vi "calibrate.vi"() -> ()   [LabVIEW 2019, in "Nano33BLE-TiltCompensationSupport.lvlib"]
uses:
  types/xyz.ctl
  types/calibrate_data.ctl
  types/xyz_array.ctl
  <vilib>/Instr/_visa.llb/VISA Configure Serial Port (Instr).vi
  Nano33BLE-TiltCompensationSupport.lvlib
  <vilib>/gmath/NI_Gmath.lvlib
panel:
  out "effective calib.":T2
  out "instructions":string
  in  "mode":bool=TRUE
  out "new config":string
  in  "initial config":string="#define OFFSET_MAG_X 0.00\n#define OFFSET_MAG_Y 0.00\n#define OFFSET_MAG_Z 0.00\n#define R_MAG 1.00\n\n#define OFFSET_ACC_X 0.00\n#define OFFSET_ACC_Y 0.00\n#define OFFSET_ACC_Z 0.00\n#define R_ACC 1.00\n\n#define OFFSET_GYR_X 0.00\n#define OFFSET_GYR_Y 0.00\n#define OFFSET_GYR_Z 0.00" caption="initial config (paste from compass-support.h)"
  in  "reset?":bool
  out "acc":cluster{dbl[], dbl[]}[](graph)
  out "mag":cluster{dbl[], dbl[]}[](graph)
  out "rates":cluster{"mag":dbl, "acc":dbl, "gyr":dbl} {"mag" format="%0.1f Hz"; "acc" format="%0.1f Hz"; "gyr" format="%0.1f Hz"}
  in  "port":refnum<visa-resource-name>="COM3"
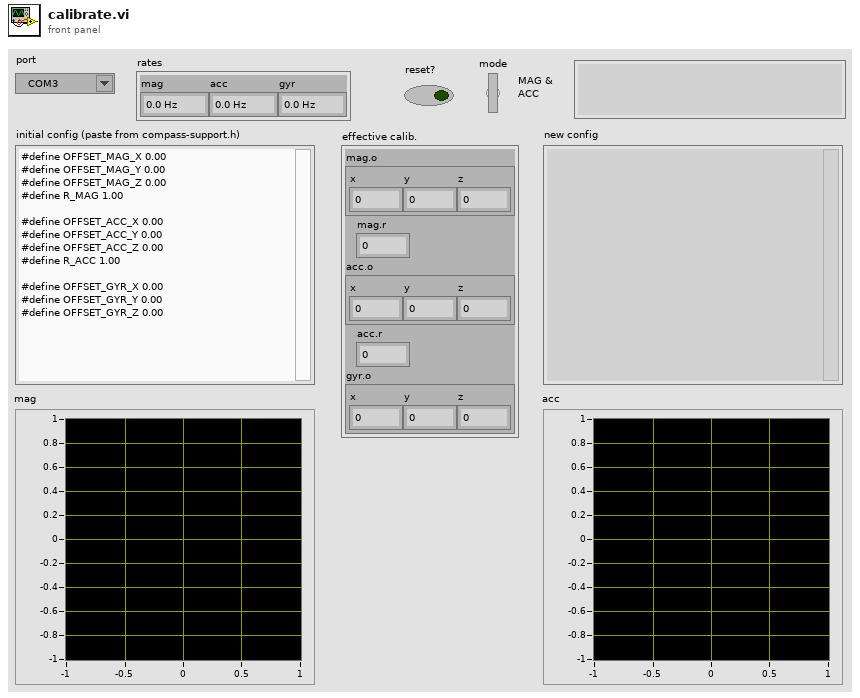
[diagram p1: front panel]
types:
  T1 = typedef "Nano33BLE-TiltCompensationSupport.lvlib/xyz.ctl" = cluster{"x":dbl, "y":dbl, "z":dbl}
  T2 = cluster{"mag.o":T1, "mag.r":dbl, "acc.o":T1, "acc.r":dbl, "gyr.o":T1}
  T3 = typedef "Nano33BLE-TiltCompensationSupport.lvlib/calibrate_data.ctl" = cluster{"mag":T4, "acc":T4, "gyr":T4, "rates":cluster{"mag":dbl, "acc":dbl, "gyr":dbl}}
  T4 = typedef "Nano33BLE-TiltCompensationSupport.lvlib/xyz_array.ctl" = cluster{"X":dbl[], "Y":dbl[], "Z":dbl[]}
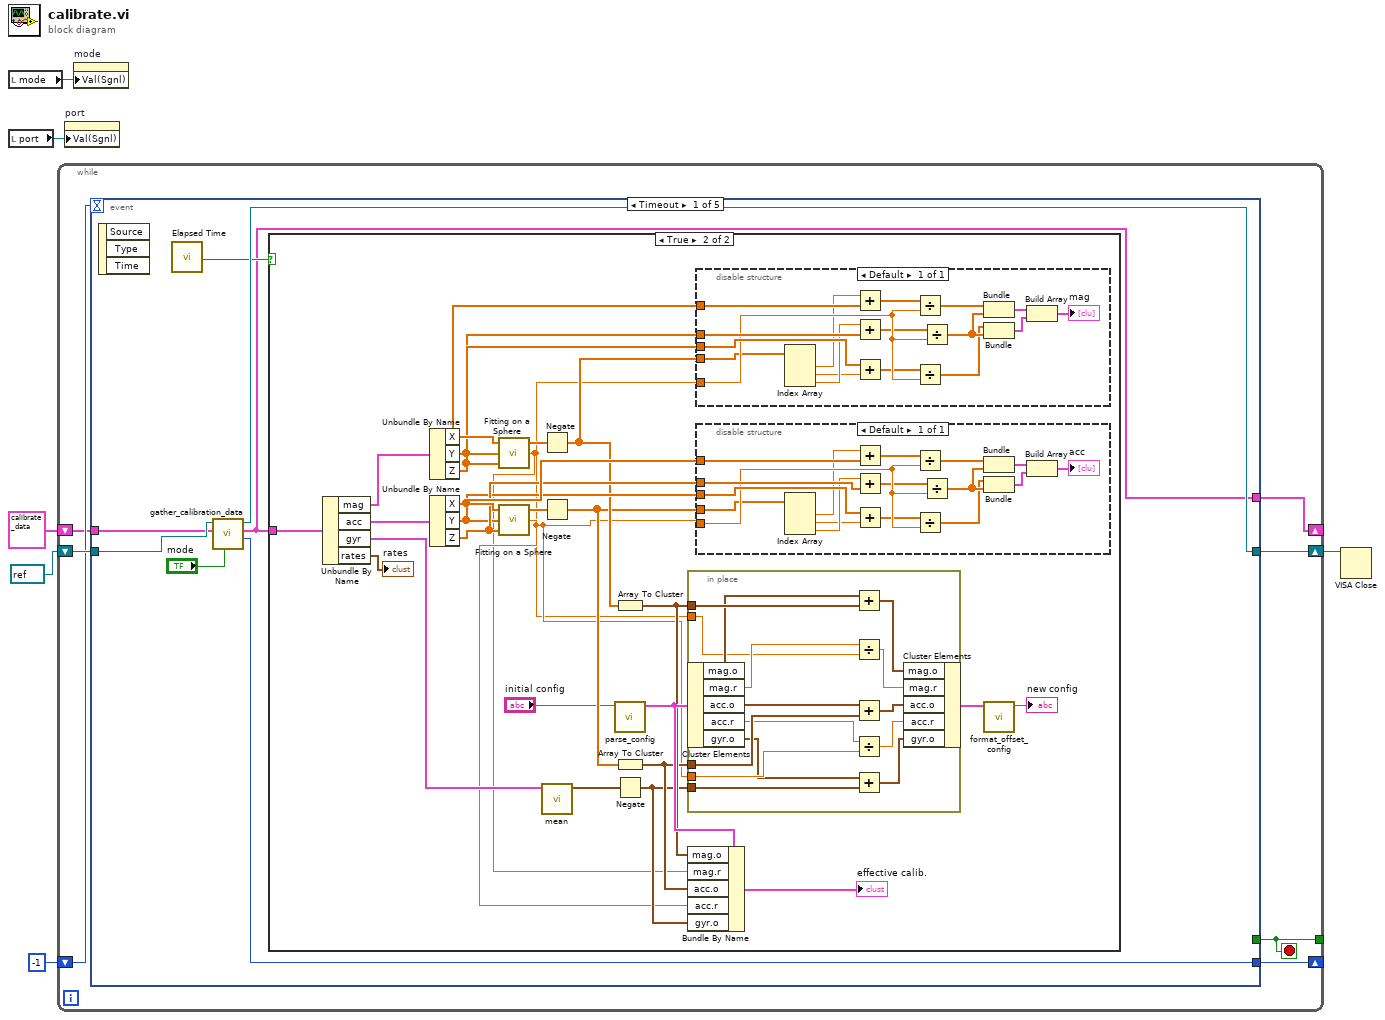
[diagram p0: block diagram]
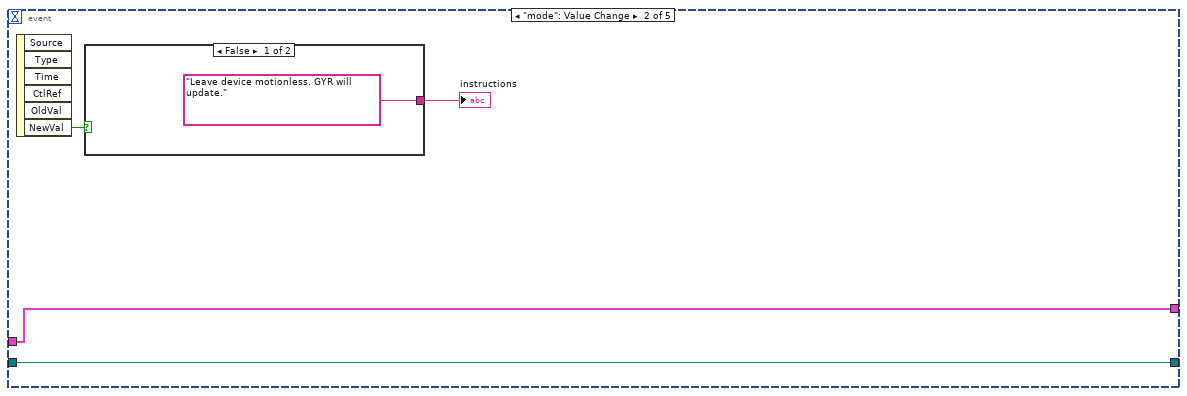
[diagram p3: hidden frame]
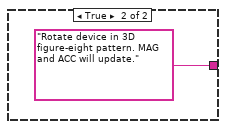
[diagram p4: hidden frame]
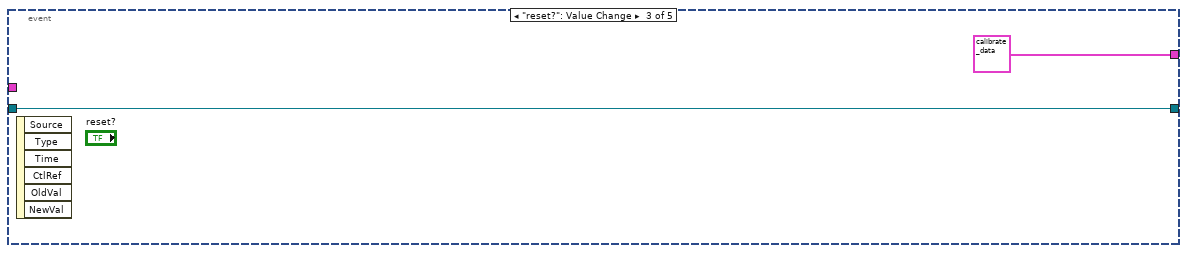
[diagram p5: hidden frame]
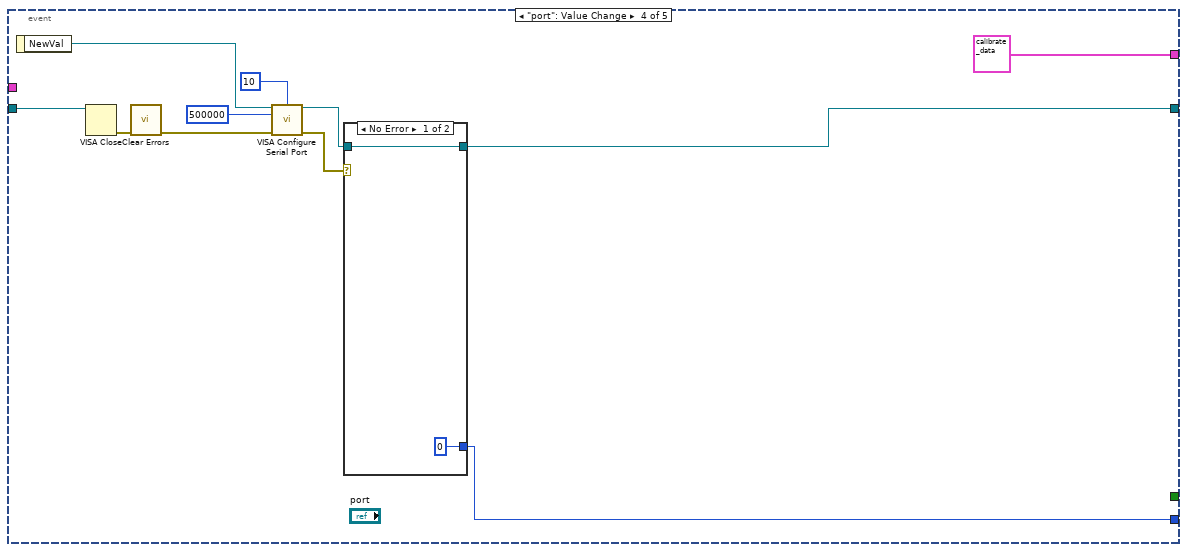
[diagram p6: hidden frame]
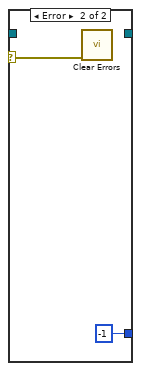
[diagram p7: hidden frame]
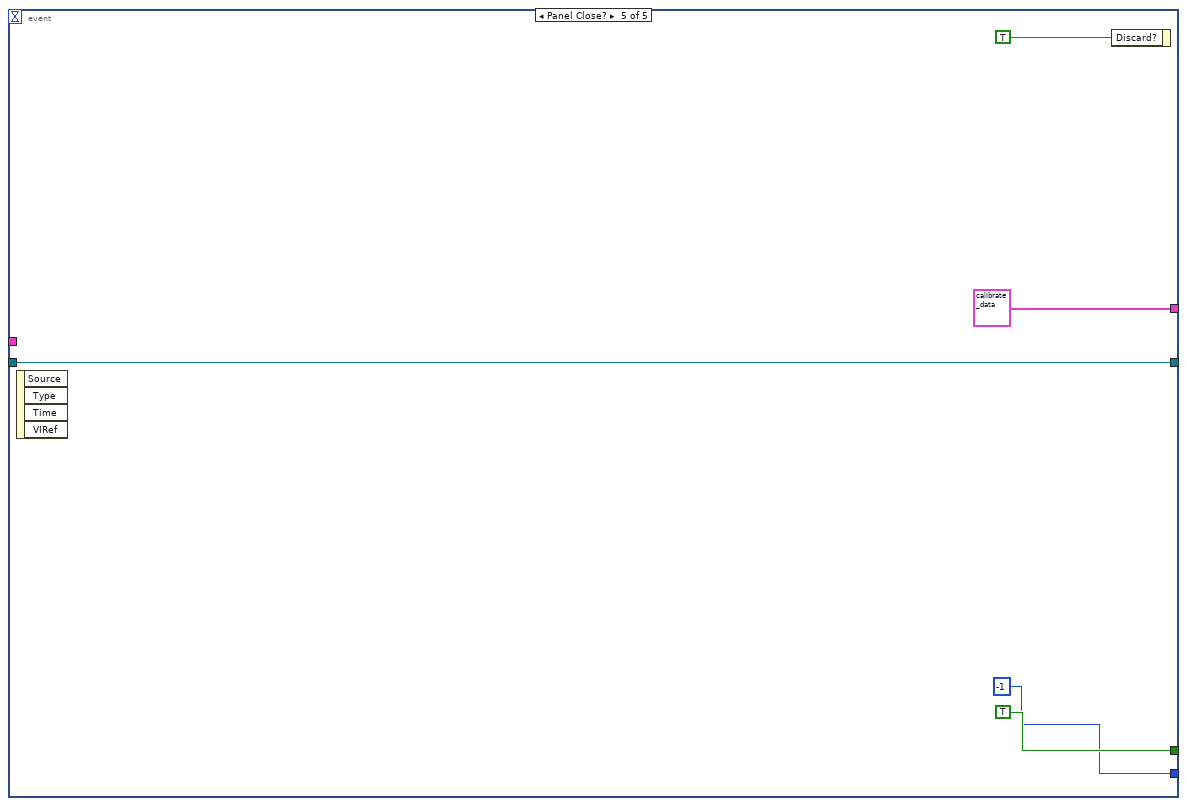
[diagram p8: hidden frame]
diagram:
  n1 = local read "mode"() -> (w1:bool)
  n2 = local read "port"() -> (w2:refnum<visa-resource-name>)
  n3 = while {
    tunnel: [w12] -> _
    shift-right: [w8] -> w3
    shift-left: refnum<visa-resource-name> refnum ("VISA resource name out") -> [w13]
    shift-right: [w9] -> _
    shift-left: -1 -> [w11]
    shift-right: [w7] -> _
    shift-left: T3 {"mag"={"X"=[], "Y"=[], "Z"=[]}, "acc"={"X"=[], "Y"=[], "Z"=[]}, "gyr"={"X"=[], "Y"=[], "Z"=[]}, "rates"={"mag"=0.0, "acc"=0.0, "gyr"=0.0}} ("data") -> [w10]
    stop <- w12 stop-if-true
    n4 = event shown="[0] Timeout" {
      selector: _ -> [_ _ _ _ _]
      dyn-events: _ -> [_ _ _ _ _]
      timeout: w11 -> [_ _ _ _ _]
      tunnel: w13 -> [w20 w96 w102 w112 w119]
      tunnel: [_ _ _ _ TRUE ("Discard?")] -> w12
      tunnel: w10 -> [w17 w99 _ _ _]
      tunnel: [w19 _ _ w108 -1] -> w9
      tunnel: [w18 w96 w102 w107 w119] -> w8
      tunnel: [w15 w99 T3 {"mag"={"X"=[], "Y"=[], "Z"=[]}, "acc"={"X"=[], "Y"=[], "Z"=[]}, "gyr"={"X"=[], "Y"=[], "Z"=[]}, "rates"={"mag"=0.0, "acc"=0.0, "gyr"=0.0}} ("data") T3 {"mag"={"X"=[], "Y"=[], "Z"=[]}, "acc"={"X"=[], "Y"=[], "Z"=[]}, "gyr"={"X"=[], "Y"=[], "Z"=[]}, "rates"={"mag"=0.0, "acc"=0.0, "gyr"=0.0}} ("data") T3 {"mag"={"X"=[], "Y"=[], "Z"=[]}, "acc"={"X"=[], "Y"=[], "Z"=[]}, "gyr"={"X"=[], "Y"=[], "Z"=[]}, "rates"={"mag"=0.0, "acc"=0.0, "gyr"=0.0}} ("data")] -> w7
      event Timeout {
        n5 = event-data() -> ()  [unwired: 1 in, 3 out]
        n6 = call "Elapsed Time"() -> ("Time has Elapsed"=w16:bool)  [unwired: 12 in, 7 out]
        n7 = call "gather_calibration_data.vi"("mode"="mode", "data in"=w17, "VISA Refnum in"=w20) -> ("next timeout (ms)"=w19:i32, "data out"=w15:T3, "VISA Refnum out"=w18:refnum<visa-resource-name>)  [unwired: 6 in]
        n8 = case shown="True" w16 {
          tunnel: w15 -> [_ w46]
          frame False {
          }
          frame True {
            n9 = Unbundle By Name(w46) -> ("mag"=w43:T4, "acc"=w42:T4, "gyr"=w45:T4, "rates"=→"rates":cluster{"mag":dbl, "acc":dbl, "gyr":dbl})
            n10 = Unbundle By Name(w43) -> ("X"=w41:dbl[], "Y"=w40:dbl[], "Z"=w39:dbl[])
            n11 = Unbundle By Name(w42) -> ("X"=w38:dbl[], "Y"=w36:dbl[], "Z"=w37:dbl[])
            n12 = call <vilib>:"Fitting on a Sphere.vi"("Z"=w39, "Y"=w40, "X"=w41) -> ("r"=w22:dbl, "x0, y0, z0"=w34:dbl[])  [unwired: 1 out]
            n13 = call <vilib>:"Fitting on a Sphere.vi"("Z"=w37, "Y"=w36, "X"=w38) -> ("r"=w23:dbl, "x0, y0, z0"=w32:dbl[])  [unwired: 1 out]
            n14 = Negate(x=w34) -> (-x=w33:dbl[])
            n15 = Negate(x=w32) -> (-x=w31:dbl[])
            n16 = call "mean.vi"("data in"=w45) -> ("xyz"=w35:T1)  [unwired: 10 in]
            n17 = Array To Cluster(array=w33) -> (cluster=w26:cluster{"[0]":dbl, "[1]":dbl, "[2]":dbl})
            n18 = call "parse_config.vi"("initial config"="initial config") -> ("config"=w27:T2)  [unwired: 10 in]
            n19 = Array To Cluster(array=w31) -> (cluster=w25:cluster{"[0]":dbl, "[1]":dbl, "[2]":dbl})
            n20 = Negate(x=w35) -> (-x=w24:T1)
            n21 = in-place {
              in-place-border: w26 -> [w61]
              in-place-border: w22 -> [w49]
              in-place-border: w25 -> [w57]
              in-place-border: w23 -> [w56]
              in-place-border: w24 -> [w52]
              n22 = in-place-cluster #1(w27) -> ("mag.o"=w50:T1, "mag.r"=w59:dbl, "acc.o"=w48:T1, "acc.r"=w47:dbl, "gyr.o"=w53:T1)
              n23 = Add(x=w50, y=w61) -> (x+y=w60:T1)
              n24 = Divide(x=w59, y=w49) -> (x/y=w58:dbl)
              n25 = Add(x=w48, y=w57) -> (x+y=w55:T1)
              n26 = Divide(x=w47, y=w56) -> (x/y=w54:dbl)
              n27 = Add(x=w53, y=w52) -> (x+y=w51:T1)
              n28 = in-place-cluster #1("mag.o"=w60, "mag.r"=w58, "acc.o"=w55, "acc.r"=w54, "gyr.o"=w51) -> (w29:T2)
            }
            n29 = Bundle By Name(cluster=w27, "mag.o"=w26, "mag.r"=w22, "acc.o"=w25, "acc.r"=w23, "gyr.o"=w24) -> (→"effective calib.":T2)
            n30 = disable-structure shown="Default" {
              disable-tunnel: w41 -> [w95]
              disable-tunnel: w40 -> [w94]
              disable-tunnel: w39 -> [w93]
              disable-tunnel: w22 -> [w92]
              disable-tunnel: w33 -> [w85]
              frame Enabled {
                n31 = Index Array(array=w85) -> (element #1=w81:dbl, element #2=w79:dbl, element #3=w80:dbl)  [unwired: 3 in]
                n32 = Add(x=w81, y=w95) -> (x+y=w84:dbl[])
                n33 = Add(x=w80, y=w93) -> (x+y=w83:dbl[])
                n34 = Add(x=w94, y=w79) -> (x+y=w82:dbl[])
                n35 = Divide(x=w84, y=w92) -> (x/y=w89:dbl[])
                n36 = Divide(x=w82, y=w92) -> (x/y=w90:dbl[])
                n37 = Divide(x=w83, y=w92) -> (x/y=w91:dbl[])
                n38 = Bundle(w89, w91) -> (w87:cluster{dbl[], dbl[]})  [unwired: 1 in]
                n39 = Bundle(w90, w91) -> (w88:cluster{dbl[], dbl[]})  [unwired: 1 in]
                n40 = Build Array(w87, w88) -> (→"mag":cluster{dbl[], dbl[]}[])
              }
            }
            n41 = disable-structure shown="Default" {
              disable-tunnel: w38 -> [w78]
              disable-tunnel: w36 -> [w77]
              disable-tunnel: w37 -> [w76]
              disable-tunnel: w23 -> [w75]
              disable-tunnel: w31 -> [w68]
              frame Enabled {
                n42 = Index Array(array=w68) -> (element #1=w64:dbl, element #2=w62:dbl, element #3=w63:dbl)  [unwired: 3 in]
                n43 = Add(x=w64, y=w78) -> (x+y=w67:dbl[])
                n44 = Add(x=w63, y=w76) -> (x+y=w66:dbl[])
                n45 = Add(x=w77, y=w62) -> (x+y=w65:dbl[])
                n46 = Divide(x=w67, y=w75) -> (x/y=w72:dbl[])
                n47 = Divide(x=w65, y=w75) -> (x/y=w73:dbl[])
                n48 = Divide(x=w66, y=w75) -> (x/y=w74:dbl[])
                n49 = Bundle(w72, w74) -> (w70:cluster{dbl[], dbl[]})  [unwired: 1 in]
                n50 = Bundle(w73, w74) -> (w71:cluster{dbl[], dbl[]})  [unwired: 1 in]
                n51 = Build Array(w70, w71) -> (→"acc":cluster{dbl[], dbl[]}[])
              }
            }
            n52 = call "format_offset_config.vi"("config"=w29) -> ("initial config"=→"new config":string)  [unwired: 10 in]
          }
        }
      }
      event "mode": Value Change {
        n53 = event-data() -> ("NewVal"=w98:bool)  [unwired: 1 in, 5 out]
        n54 = case shown="False" w98 {
          tunnel: ["Leave device motionless. GYR will update." "Rotate device in 3D figure-eight pattern. MAG and ACC will update."] -> w97
          frame False {
          }
          frame True {
          }
        }
        "instructions" <- w97
      }
      event "reset?": Value Change {
        n55 = event-data() -> ()  [unwired: 1 in, 6 out]
      }
      event "port": Value Change {
        n56 = event-data() -> ("NewVal"=w104:refnum<visa-resource-name>)  [unwired: 1 in]
        n57 = VISA Close(VISA resource name=w112) -> (error out=w111:errorcluster)  [unwired: 1 in]
        n58 = call <vilib>:"Clear Errors.vi"("error in (no error)"=w111) -> ("error out"=w110:errorcluster)  [unwired: 5 in, 1 out]
        n59 = call-poly "VISA Configure Serial Port"("VISA resource name"=w104, "termination char\n(0xA = '\\n' = LF)"=u8 10 ("termination char\n(0xA = '\\n' = LF)"), "baud rate (9600)"=u32 500000, "error in (no error)"=w110) -> ("VISA resource name out"=w106:refnum<visa-resource-name>, "error out"=w109:errorcluster)  [unwired: 10 in]
        n60 = case shown="No Error" w109 {
          selector: w109 -> [_ w118]
          tunnel: [0 -1] -> w108
          tunnel: [w115 _] -> w107
          tunnel: w106 -> [w115 _]
          frame No Error {
          }
          frame Error {
            n61 = call <vilib>:"Clear Errors.vi"("error in (no error)"=w118) -> ()  [unwired: 5 in, 2 out]
          }
        }
      }
      event Panel Close? {
        n62 = event-data() -> ()  [unwired: 1 in, 4 out]
        n63 = event-data("Discard?"=TRUE) -> ()  [unwired: 1 in, 1 out]
      }
    }
  }
  n64 = property on="port" class="VISAName"("Val(Sgnl)"=w2) -> ()  [unwired: 2 in, 2 out]
  n65 = property on="mode" class="Bool (strict)"("Val(Sgnl)"=w1) -> ()  [unwired: 2 in, 2 out]
  n66 = VISA Close(VISA resource name=w3) -> ()  [unwired: 1 in, 1 out]
